vi "Inverse Error Function_Iteration.vi"(11 "x":dbl) -> (3 "erfinv(x)":dbl)   [LabVIEW 2020, in "NI_AAL_MathFunc.lvlib"]
uses:
  <vilib>/gmath/NI_AAL_MathFunc.lvlib
  <vilib>/gmath/NI_Gmath.lvlib
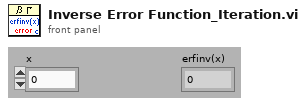
[diagram p1: front panel]
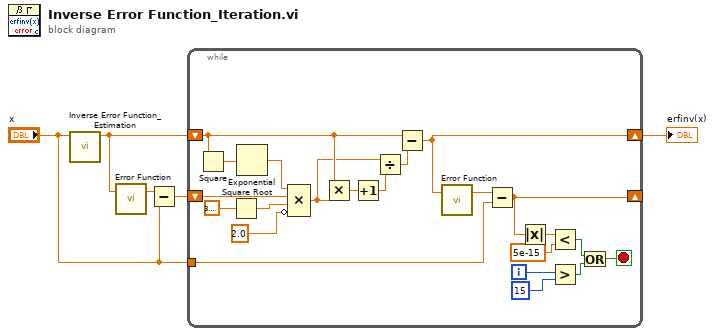
[diagram p0: block diagram]
diagram:
  n1 = call <vilib>:"Inverse Error Function_Estimation.vi"("x"="x") -> ("erf^-1(x)"=w3:dbl)  [unwired: 10 out]
  n2 = call <vilib>:"Error Function.vi"("x"=w3) -> ("erf(x)"=w2:dbl)  [unwired: 2 out]
  n3 = Subtract(x=w2, y="x") -> (x-y=w1:dbl)
  n4 = while {
    shift-right: [w24] -> w4
    shift-left: w3 -> [w21]
    shift-right: [w16] -> _
    shift-left: w1 -> [w18]
    tunnel: "x" -> [w22]
    i -> [w6]
    stop <- w10 stop-if-true
    n5 = Square(x=w21) -> (x^2=w17:dbl)
    n6 = Square Root(x=3.141592653589793) -> (sqrt(x)=w8:dbl)
    n7 = Exponential(1:w17) -> (0:w19:dbl)
    n8 = Compound Arithmetic op=MULTIPLY(w19, w18, w8, invert 2.0 ("value")) -> (w20:dbl)
    n9 = Multiply(x=w21, y=w20) -> (x*y=w27:dbl)
    n10 = Increment(x=w27) -> (x+1=w26:dbl)
    n11 = Divide(x=w20, y=w26) -> (x/y=w25:dbl)
    n12 = Subtract(x=w21, y=w25) -> (x-y=w24:dbl)
    n13 = call <vilib>:"Error Function.vi"("x"=w24) -> ("erf(x)"=w23:dbl)  [unwired: 2 out]
    n14 = Subtract(x=w23, y=w22) -> (x-y=w16:dbl)
    n15 = Absolute Value(x=w16) -> (abs(x)=w15:dbl)
    n16 = Less?(x=w15, y=5e-15) -> (x < y?=w12:bool)
    n17 = Greater?(x=w6, y=15) -> (0:w11:bool)
    n18 = Or(x=w12, y=w11) -> (x .or. y?=w10:bool)
  }
  "erfinv(x)" <- w4
